vi "sub_VI_Fourier_series_disp.vi"(10 "del t":dbl, 11 "x,i":dbl[](array[numeric])=[1.388528617422219e-06, 1.0215603399606325e-05, 2.122465172345392e-05, 2.9975433724460983e-05, 3.867281077864411e-05, 4.72938950516502e-05, 5.581579870912612e-05, 6.427666814166041e-05, 7.25773227337229e-05, 8.279292613332924e-05, 9.083418526938979e-05, 9.869234173062542e-05, 0.00010644368829821318, 0.00011401193219097605, 0.00012141233196514943, 0.00013043013870027613, 0.0001374490745685643, 0.000144246761371439, 0.00015087660405572418, 0.00015725468056212516, 0.0001634343958374658, 0.00017082716633352147, 0.0001764575735843874, 0.00018186673176983988, 0.0001870088652211727, 0.0001918916032165036, 0.0001964996871995971, 0.00020187832827257878, 0.00020583792361566743, 0.00020953049422463643, 0.00021290263515266178, 0.00021600012206844982, 0.00021877717930329427, 0.00022182889055037604, 0.00022393457131086248, 0.00022571219311228765, 0.0002271693852327692, 0.00022831377695042488, 0.00022915299754337239, 0.0002297175641240825, 0.0002298320032958481, 0.00022961075423043466, 0.00022907670476219534, 0.0002281917085005416, 0.00022703968750476824, 0.00022510185086287127, 0.00022320216061156285, 0.0002209972992355463, 0.0002184796374567038, 0.0002156262874406823, 0.00021249065413430574, 0.0002081495948853319, 0.00020434258510459733, 0.0002002532920335077, 0.00019590460350641617, 0.00019124311457649872, 0.00018631460091246161, 0.00017981445595617737, 0.00017432137571143013, 0.00016859178784503406, 0.00016261043380075372, 0.00015642308924729536, 0.00014998397851595277, 0.00014168332392389027, 0.00013484749073042703, 0.0001278056670277858, 0.00012060362848467275, 0.0001132413751010879, 0.00010574179471138436, 9.618230922990063e-05, 8.836229915925353e-05, 8.042784991684085e-05, 7.23713322245449e-05, 6.420800463860107e-05, 5.5907350046538575e-05, 4.540183407845948e-05, 3.689518897721896e-05, 2.8358026763507628e-05, 1.976745960297236e-05, 1.1115858217495457e-05, 2.4795153882539626e-06, -8.315913148297907e-06, -1.6944626699421696e-05, -2.5519935303721554e-05, -3.404183896119748e-05, -4.248744983749636e-05, -5.08643972107359e-05, -6.122495689457861e-05, -6.940354303675784e-05, -7.74524314509361e-05, -8.537925141523107e-05, -9.318400292964277e-05, -0.00010089720310664201, -0.00011030410302577168, -0.00011762821001876798, -0.00012482261928376334, -0.00013182629659581606, -0.0001386392419549262, -0.00014523093824862286, -0.00015323405099409488, -0.00015937561987884702, -0.00016531882753253882, -0.0001710102690083464, -0.00017646520286250509, -0.00018166837053877957, -0.0001878251979797671, -0.00019247142835344914, -0.0001968277461586584, -0.000200917039229748, -0.00020473167828860027, -0.00020824114622274435, -0.00021223125867830377, -0.00021507697941620756, -0.0002176327875856386, -0.00021989105390847913, -0.00022182126127225833, -0.0002234691853456825, -0.00022507896302851815, -0.0002259944764026427, -0.00022660481865205908, -0.00022687947266429644, -0.0002268260677174725, -0.0002264827502021758, -0.00022559775394052206, -0.00022453728428216115, -0.0002231106092741504, -0.00022140928025390233, -0.00021936463371835752, -0.0002169995575018691, -0.0002135816409051375, -0.00021052992965805566, -0.0002071577887300303, -0.00020349573523353214, -0.0001995285106123258, -0.0001952713734226467, -0.00018956467339060373, -0.00018468193539527284, -0.0001795321726658223, -0.00017415353159284063, -0.00016846209011703306, -0.0001625570288539298, -0.00015486671651128366, -0.00014841234722370565, -0.00014176724598318502, -0.00013492378351160408, -0.0001278590719746097, -0.00012059599920655504, -0.00011128065062483784, -0.00010359796756030941, -9.580847460213311e-05, -8.784350824724962e-05, -7.973358560812974e-05, -7.149396524100888e-05, -6.105711277598912e-05, -5.258098478721941e-05, -4.401330546103726e-05, -3.539222118803118e-05, -2.670247341196575e-05, -1.7974579245311805e-05, -7.0036773120527314e-06]) -> (0 "clipped array":dbl[](array[numeric]), 3 "outputs":T1)   [LabVIEW 2018]
uses:
  Fourier Outputs.ctl
panel:
  out "a":dbl
  out "Waveform Chart 2":dbl[](graph)
  out "Waveform Chart":dbl[](graph)
  out "t,i":dbl[](array[numeric])
  out "b":dbl
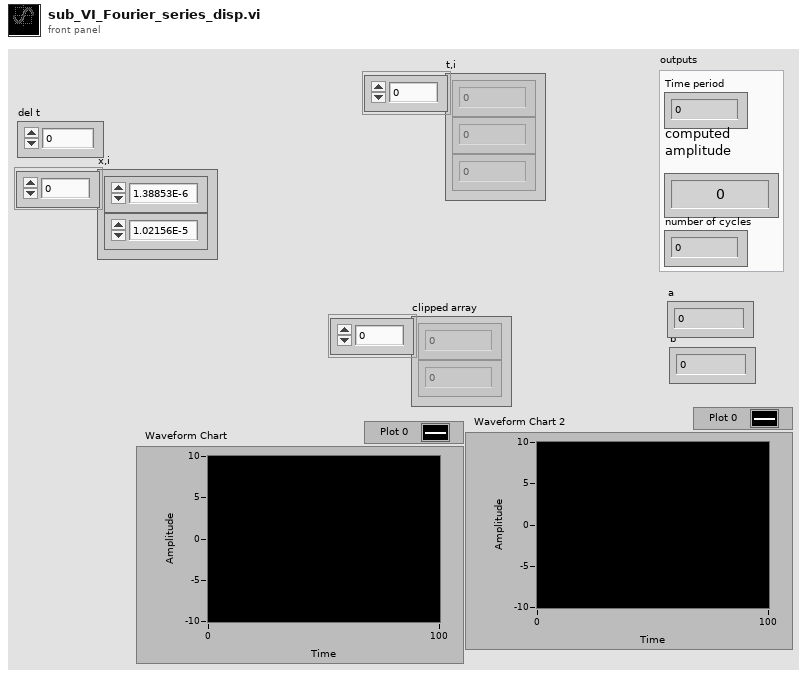
[diagram p1: front panel]
types:
  T1 = typedef "Fourier Outputs.ctl" = cluster{"Time period":dbl, "computed \namplitude":dbl, "number of cycles":dbl}
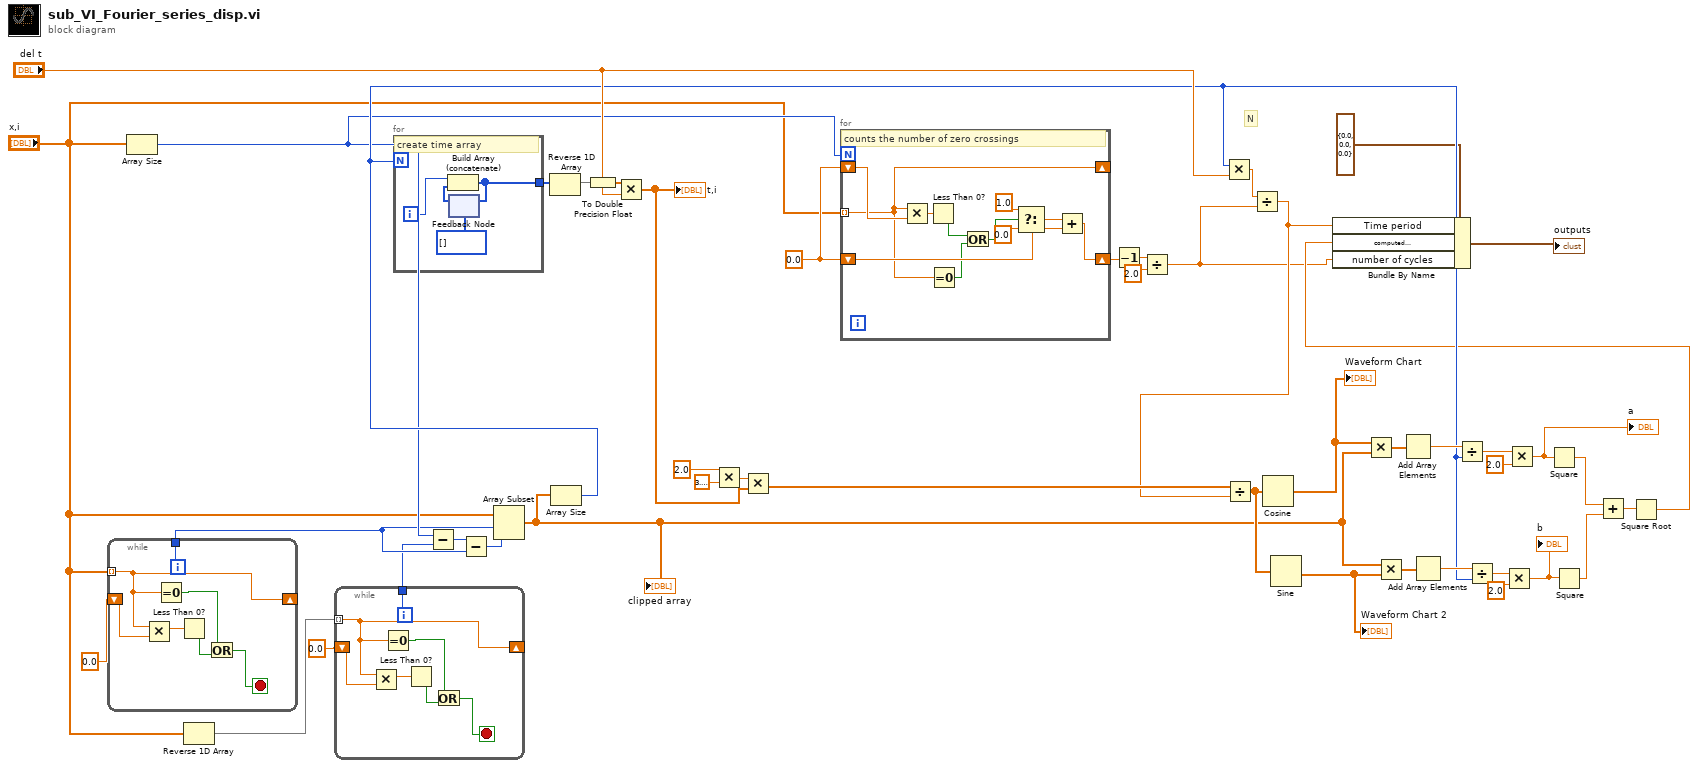
[diagram p0: block diagram]
diagram:
  w26 = 0.0 ("Numeric Control")
  # "N"
  n1 = while {
    tunnel: "x,i" -> [w50] mode=indexing
    shift-right: [w50] -> _
    shift-left: 0.0 -> [w53]
    tunnel: [w52] -> w12
    i -> [w52]
    stop <- w49 stop-if-true
    n2 = Multiply(x=w50, y=w53) -> (x*y=w51:dbl)
    n3 = Equal To 0?(x=w50) -> (x = 0?=w48:bool)
    n4 = Less Than 0?(x=w51) -> (x < 0?=w47:bool)
    n5 = Or(x=w48, y=w47) -> (x .or. y?=w49:bool)
  }
  n6 = Array Size(array="x,i") -> (size(s)=w14:i32)
  n7 = Reverse 1D Array(array="x,i") -> (reversed array=w8:dbl[])
  n8 = while {
    tunnel: w8 -> [w57] mode=indexing
    shift-right: [w57] -> _
    shift-left: 0.0 -> [w60]
    tunnel: [w59] -> w7
    i -> [w59]
    stop <- w56 stop-if-true
    n9 = Multiply(x=w57, y=w60) -> (x*y=w58:dbl)
    n10 = Equal To 0?(x=w57) -> (x = 0?=w55:bool)
    n11 = Less Than 0?(x=w58) -> (x < 0?=w54:bool)
    n12 = Or(x=w55, y=w54) -> (x .or. y?=w56:bool)
  }
  n13 = Subtract(x=w14, y=w7) -> (x-y=w21:i32)
  n14 = Subtract(x=w21, y=w12) -> (x-y=w20:i32)
  n15 = Array Subset(array="x,i", index=w12, length=w20) -> (w16:dbl[])
  "clipped array" <- w16
  n16 = Array Size(array=w16) -> (size(s)=w15:i32)
  n17 = for {
    N: w15 -> [_]
    tunnel: [w61] -> w46
    i -> [w64]
    # "create time array"
    n18 = feedback #1(i32[] []) -> (w63:i32[])
    n19 = Build Array (concatenate)(w64, w63) -> (w61:i32[])
    n20 = feedback-in #1(w61) -> ()
  }
  n21 = Reverse 1D Array(array=w46) -> (reversed array=w24:i32[])
  n22 = To Double Precision Float(number=w24) -> (double precision float=w25:dbl[])
  n23 = Multiply(x=w25, y="del t") -> (x*y=w19:dbl[])
  "t,i" <- w19
  n24 = Multiply(x=2.0, y=3.141592653589793) -> (x*y=w31:dbl)
  n25 = Multiply(x=w31, y=w19) -> (x*y=w32:dbl[])
  n26 = for {
    N: w14 -> [_]
    tunnel: "x,i" -> [w68] mode=indexing
    shift-right: [w68] -> _
    shift-left: w26 -> [w72]
    shift-right: [w70] -> w17
    shift-left: w26 -> [w71]
    # "counts the number of zero crossings"
    n27 = Multiply(x=w68, y=w72) -> (x*y=w69:dbl)
    n28 = Less Than 0?(x=w69) -> (x < 0?=w66:bool)
    n29 = Equal To 0?(x=w68) -> (x = 0?=w67:bool)
    n30 = Or(x=w66, y=w67) -> (x .or. y?=w65:bool)
    n31 = Select(t=1.0, s=w65, f=0.0) -> (s? t:f=w73:dbl)
    n32 = Add(x=w73, y=w71) -> (x+y=w70:dbl)
  }
  n33 = Decrement(x=w17) -> (x-1=w18:dbl)
  n34 = Divide(x=w18, y=2.0) -> (x/y=w2:dbl)
  n35 = Multiply(x=w15, y="del t") -> (x*y=w45:dbl)
  n36 = Divide(x=w45, y=w2) -> (x/y=w6:dbl)
  n37 = Divide(x=w32, y=w6) -> (x/y=w36:dbl[])
  n38 = Cosine(x=w36) -> (cos(x)=w11:dbl[])
  "Waveform Chart" <- w11
  n39 = Sine(x=w36) -> (sin(x)=w10:dbl[])
  "Waveform Chart 2" <- w10
  n40 = Multiply(x=w11, y=w16) -> (x*y=w33:dbl[])
  n41 = Multiply(x=w16, y=w10) -> (x*y=w37:dbl[])
  n42 = Add Array Elements(numeric array=w33) -> (sum=w34:dbl)
  n43 = Add Array Elements(numeric array=w37) -> (sum=w38:dbl)
  n44 = Divide(x=w34, y=w15) -> (x/y=w35:dbl)
  n45 = Divide(x=w38, y=w15) -> (x/y=w39:dbl)
  n46 = Multiply(x=w39, y=2.0) -> (x*y=w40:dbl)
  "b" <- w40
  n47 = Multiply(x=w35, y=2.0) -> (x*y=w1:dbl)
  "a" <- w1
  n48 = Square(x=w1) -> (x^2=w41:dbl)
  n49 = Square(x=w40) -> (x^2=w42:dbl)
  n50 = Add(x=w41, y=w42) -> (x+y=w43:dbl)
  n51 = Square Root(x=w43) -> (sqrt(x)=w3:dbl)
  n52 = Bundle By Name(cluster=T1 {"Time period"=0.0, "computed \namplitude"=0.0, "number of cycles"=0.0} ("outputs 2"), "Time period"=w6, "computed \namplitude"=w3, "number of cycles"=w2) -> (→"outputs":T1)
